vi "unloadSubPanelVi.vi"(8 "error in (no error)":errorcluster, 11 "ActionEditor in":refnum<class "ActionEditor.lvclass">) -> (0 "error out":errorcluster, 1 "editing":bool, 2 "ScriptEvent":refnum<class "ScriptEvent.lvclass">, 3 "ActionEditor out":refnum<class "ActionEditor.lvclass">)   [LabVIEW 2011, in "Views.lvlib" / "ScriptEditor.lvlib" / "ActionEditor.lvclass"]
uses:
  ActionEditor.lvclass
  Tools/Scripting/ScriptingEvent/ScriptEvent.lvclass
  ActionEditor.lvclass/ActionEditor.ctl
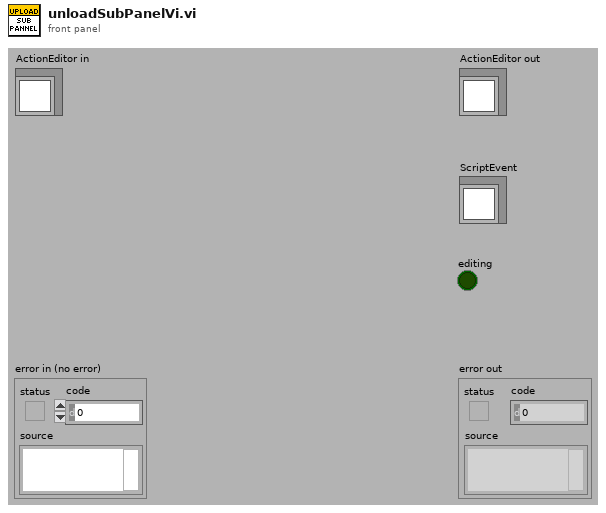
[diagram p1: front panel]
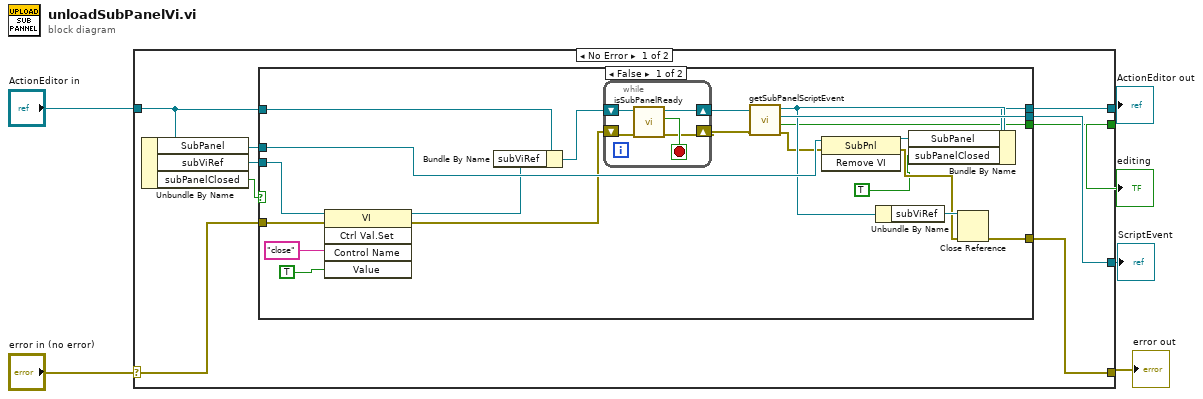
[diagram p0: block diagram]
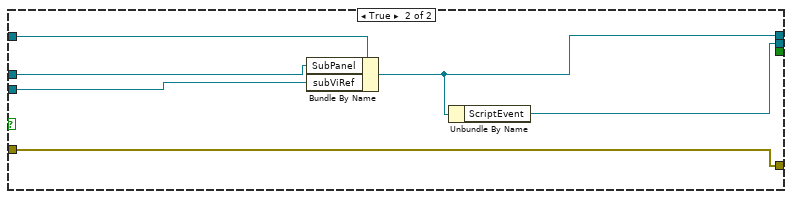
[diagram p2: hidden frame]
diagram:
  n1 = case shown="No Error" "error in (no error)" {
    selector: "error in (no error)" -> [w12 w49]
    tunnel: [w13 w49] -> w5
    tunnel: [w10 w48] -> w3
    tunnel: "ActionEditor in" -> [w15 w48]
    tunnel: [w14 _] -> w2
    tunnel: [w9 _] -> w1
    frame No Error {
      n2 = Unbundle By Name(w15) -> ("SubPanel"=w11:refnum<vi>, "subViRef"=w7:refnum<vi>, "subPanelClosed"=w8:bool)
      n3 = case shown="False" w8 {
        tunnel: w7 -> [w34 w45]
        tunnel: w15 -> [w33 w47]
        tunnel: [w29 w43] -> w14
        tunnel: [w27 w42] -> w13
        tunnel: w12 -> [w26 w42]
        tunnel: w11 -> [w25 w46]
        tunnel: [w22 w44] -> w10
        tunnel: [w17 _] -> w9
        frame False {
          n4 = invoke class="VI" method="Ctrl Val.Set"(reference=w34, error in=w26, "Control Name"="close", "Value"=TRUE) -> (reference out=w19:refnum<vi>, error out=w18:errorcluster)  [unwired: 1 in, 3 out]
          n5 = Bundle By Name(cluster=w33, "subViRef"=w19) -> (w32:refnum<class "ActionEditor.lvclass">)
          n6 = while {
            shift-right: [w37] -> w30
            shift-left: w18 -> [w39]
            shift-right: [w40] -> w31
            shift-left: w32 -> [w41]
            stop <- w38 stop-if-true
            n7 = call "isSubPanelReady.vi"("error in (no error)"=w39, "ActionEditor in"=w41) -> ("error out"=w37:errorcluster, "ready?"=w38:bool, "ActionEditor out"=w40:refnum<class "ActionEditor.lvclass">)  [unwired: 7 in]
          }
          n8 = call "getSubPanelScriptEvent.vi"("error in (no error)"=w30, "ActionEditor in"=w31) -> ("error out"=w21:errorcluster, "editing"=w17:bool, "ScriptEvent"=w29:refnum<class "ScriptEvent.lvclass">, "ActionEditor out"=w23:refnum<class "ActionEditor.lvclass">)  [unwired: 6 in]
          n9 = invoke class="SubPnl" method="Remove VI"(reference=w25, error in=w21) -> (reference out=w24:refnum<vi>, error out=w20:errorcluster)  [unwired: 1 in, 1 out]
          n10 = Unbundle By Name(w23) -> ("subViRef"=w28:refnum<vi>)
          n11 = Bundle By Name(cluster=w23, "SubPanel"=w24, "subPanelClosed"=TRUE) -> (w22:refnum<class "ActionEditor.lvclass">)
          n12 = Close Reference(reference=w28, error in (no error)=w20) -> (error out=w27:errorcluster)
        }
        frame True {
          n13 = Bundle By Name(cluster=w47, "SubPanel"=w46, "subViRef"=w45) -> (w44:refnum<class "ActionEditor.lvclass">)
          n14 = Unbundle By Name(w44) -> ("ScriptEvent"=w43:refnum<class "ScriptEvent.lvclass">)
        }
      }
    }
    frame Error {
    }
  }
  "error out" <- w5
  "ActionEditor out" <- w3
  "ScriptEvent" <- w2
  "editing" <- w1
